vi "Controlword.vi"(8 "error in":errorcluster, 9 "W/R":enum16{"Write", "Read"}(ring), 10 "Data":u16 format="%x", 11 "Motor Base in":refnum<class "Motor Base.lvclass">) -> (0 "error out":errorcluster, 2 "Data":u16, 3 "Motor Base out":refnum<class "Motor Base.lvclass">)   [LabVIEW 2016, in "Motor Base.lvlib" / "Motor Base.lvclass"]
uses:
  Motor Base.lvclass
  Data Type.ctl
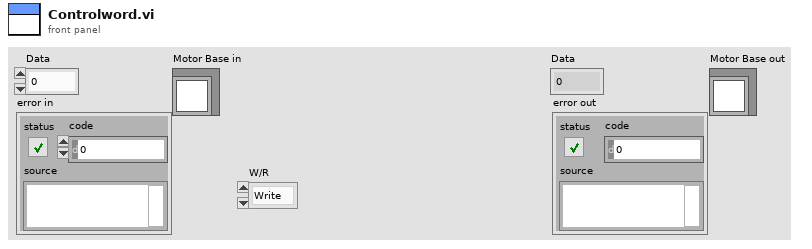
[diagram p1: front panel]
types:
  T1 = typedef "Motor Base.lvlib/Motor Base.lvclass/Data Type.ctl" = enum16{"BOOL", "I16", "I32", "I8", "OS", "U16", "U32", "U8", "VS"}
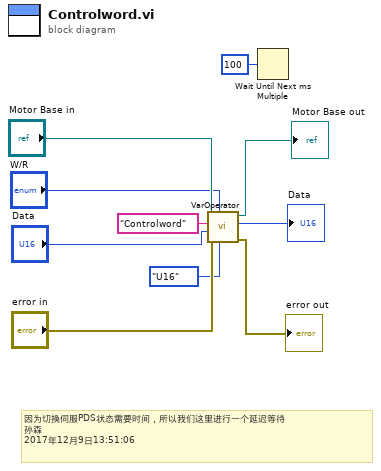
[diagram p0: block diagram]
diagram:
  # "因为切换伺服PDS状态需要时间，所以我们这里进行一个延迟等待\n孙森\n2017年12月9日13:51:06"
  n1 = call-dynamic "VarOperator.vi"("Data Type"=Data_Type."U16", "ro/w/r"="W/R", "error in"="error in", "Data"="Data", "PDO Name"="Controlword", "Motor Base in"="Motor Base in") -> ("error out"=→"error out":errorcluster, "Data"=→"Data":i64, "Motor Base out"=→"Motor Base out":refnum<class "Motor Base.lvclass">)  [unwired: 1 in, 2 out]
  n2 = Wait Until Next ms Multiple(millisecond multiple=u32 100) -> ()  [unwired: 1 out]
